vi "Convert Color to Greyscale Index.vi"(11 "Color in":u32(colorbox)) -> (3 "Grey Scale Index (0-255)":u8)   [LabVIEW 2015, in "ColorSelector.lvclass"]
doc: "This VI will convert the RGB Color Scale to the Grey Color Scale. It calculates the tone of the color. See Wikipedia article: https://en.wikipedia.org/wiki/Luma_(video).\n<b> </b> <b> </b>\n©2017 Q Software Innovations, LLC (QSI)\nwritten by Quentin Alldredge\nproduced in LabVIEW 2015\n\nsupport@qsoftwareinnovations.com\nwww.qsoftwareinnovations.com\n\nAll rights reserved.\n\nRedistribution and use in source and binary forms, with or without modification, are permitted provided that the following conditions are met:\n\n * Redistributions of source code must retain the above copyright notice, this list of conditions and the following disclaimer.\n * Redistributions in binary form must reproduce the above copyright notice, this list of conditions and the following disclaimer in the documentation and/or other materials provided with the distribution.\n * Neither the name of Q Software Innovations, LLC. nor the names of its contributors may be used to endorse or promote products derived from this software without specific prior written permission.\n\nTHIS SOFTWARE IS PROVIDED BY THE COPYRIGHT HOLDERS AND CONTRIBUTORS \"AS IS\" AND ANY EXPRESS OR IMPLIED WARRANTIES, INCLUDING, BUT NOT LIMITED TO, THE IMPLIED WARRANTIES OF MERCHANTABILITY AND FITNESS FOR A PARTICULAR PURPOSE ARE DISCLAIMED. IN NO EVENT SHALL THE COPYRIGHT OWNER OR CONTRIBUTORS BE LIABLE FOR ANY DIRECT, INDIRECT, INCIDENTAL, SPECIAL, EXEMPLARY, OR CONSEQUENTIAL DAMAGES (INCLUDING, BUT NOT LIMITED TO, PROCUREMENT OF SUBSTITUTE GOODS OR SERVICES; LOSS OF USE, DATA, OR PROFITS; OR BUSINESS INTERRUPTION) HOWEVER CAUSED AND ON ANY THEORY OF LIABILITY, WHETHER IN CONTRACT, STRICT LIABILITY, OR TORT (INCLUDING NEGLIGENCE OR OTHERWISE) ARISING IN ANY WAY OUT OF THE USE OF THIS SOFTWARE, EVEN IF ADVISED OF THE POSSIBILITY OF SUCH DAMAGE."
uses:
  ColorSelector.lvclass
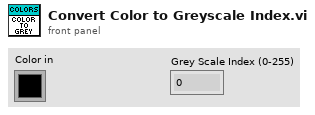
[diagram p1: front panel]
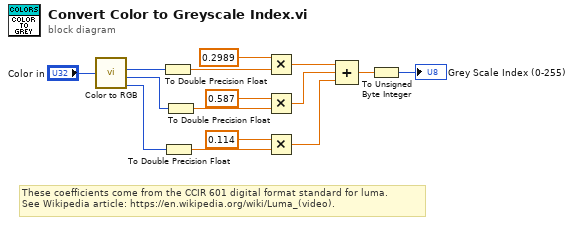
[diagram p0: block diagram]
diagram:
  # "These coefficients come from the CCIR 601 digital format standard for luma.\nSee Wikipedia article: https://en.wikipedia.org/wiki/Luma_(video)."
  n1 = call <vilib>:"Color to RGB.vi"("Color"="Color in") -> ("R"=w7:u8, "G"=w8:u8, "B"=w9:u8)  [unwired: 1 out]
  n2 = To Double Precision Float(number=w7) -> (double precision float=w6:dbl)
  n3 = To Double Precision Float(number=w9) -> (double precision float=w4:dbl)
  n4 = To Double Precision Float(number=w8) -> (double precision float=w5:dbl)
  n5 = Multiply(x=0.2989, y=w6) -> (x*y=w15:dbl)
  n6 = Multiply(x=0.587, y=w5) -> (x*y=w14:dbl)
  n7 = Multiply(x=0.114, y=w4) -> (x*y=w13:dbl)
  n8 = Compound Arithmetic op=ADD(w15, w14, w13) -> (w3:dbl)
  n9 = To Unsigned Byte Integer(number=w3) -> (unsigned 8bit integer=→"Grey Scale Index (0-255)":u8)
